vi "Choreo_TrajectoryDifferential_SampleAt.vi"(9 "MirrorForRedAlliance":bool, 10 "TimeStamp":dbl, 11 "ChoreoTrajectoryDifferential":T2) -> (3 "ChoreoDifferentialSample":T1={"timestamp"=-999.0, "x"=0.0, "y"=0.0, "heading"=0.0, "velocityL"=0.0, "velocityR"=0.0, "angularVelocity"=0.0, "accelL"=0.0, "accelR"=0.0, "accelAngular"=0.0, "forceL"=0.0, "forceR"=0.0})   [LabVIEW 2019, in "ChoreoLib.lvlib"]
doc: "Return an interpolated sample of the trajectory at the given timestamp.\n\nInputs: \n - ChoreoTrajectory - cluster - The trajectory to sample.\n - timestamp - double - The timestamp of this sample relative to the beginning of the trajectory.\n - mirrorForRedAlliance - boolean - whether or not to return the sample as mirrored across the field midline (as in 2023). (Optional. Default: false )\n\nOutputs:\n - ChoreoTrajectoryState - cluster - The ChoreoTrajectoryState at the given time."
uses:
  ChoreoLib.lvlib
  TypeDef/ChoreoEventMarker.ctl
  TypeDef/ChoreoDifferentialSample.ctl
  TypeDef/ChoreoTrajectoryDifferential.ctl
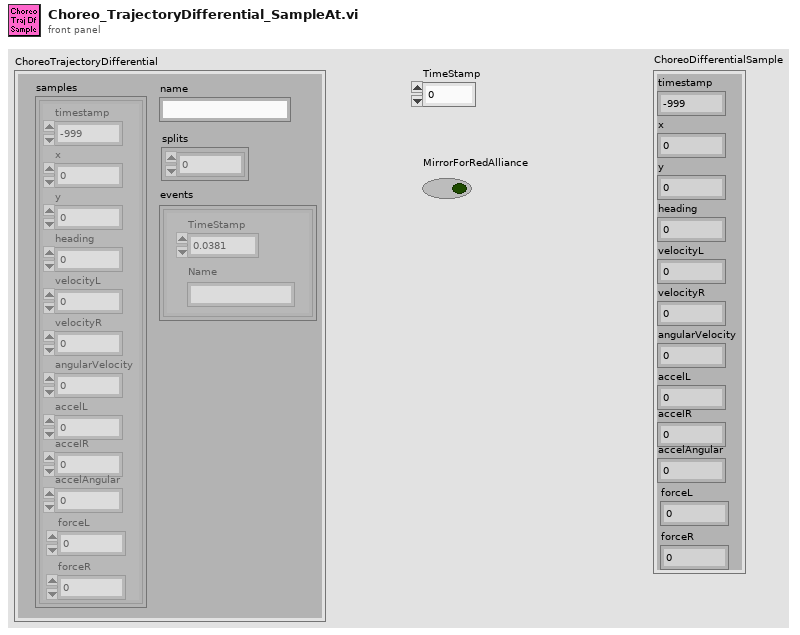
[diagram p1: front panel]
types:
  T1 = typedef "ChoreoLib.lvlib/ChoreoDifferentialSample.ctl" = cluster{"timestamp":dbl, "x":dbl, "y":dbl, "heading":dbl, "velocityL":dbl, "velocityR":dbl, "angularVelocity":dbl, "accelL":dbl, "accelR":dbl, "accelAngular":dbl, "forceL":dbl, "forceR":dbl}
  T2 = typedef "ChoreoLib.lvlib/ChoreoTrajectoryDifferential.ctl" = cluster{"name":string, "samples":T1[], "splits":i32[], "events":T3[]}
  T3 = typedef "ChoreoLib.lvlib/ChoreoEventMarker.ctl" = cluster{"TimeStamp":dbl, "Name":string}
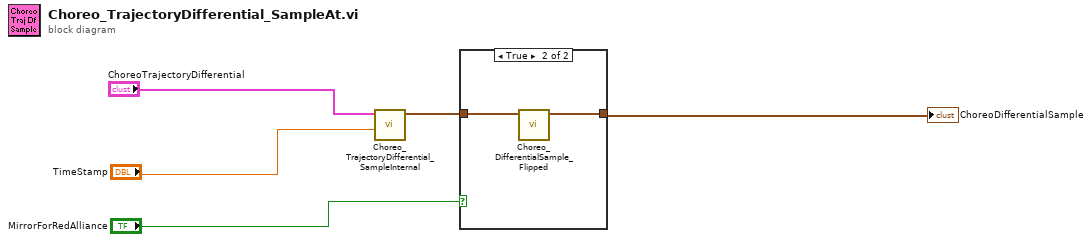
[diagram p0: block diagram]
diagram:
  n1 = call "Choreo_TrajectoryDifferential_SampleInternal.vi"("TimeStamp"="TimeStamp", "ChoreoTrajectoryDifferential"="ChoreoTrajectoryDifferential") -> ("ChoreoSwerveSample"=w2:T1)  [unwired: 9 in]
  n2 = case shown="True" "MirrorForRedAlliance" {
    tunnel: w2 -> [w6 w8]
    tunnel: [w6 w7] -> w1
    frame False {
    }
    frame True {
      n3 = call "Choreo_DifferentialSample_Flipped.vi"("ChoreoDifferentialSample"=w8) -> ("FlippedDifferentialSample"=w7:T1)  [unwired: 10 in]
    }
  }
  "ChoreoDifferentialSample" <- w1
